vi "Read Class Path.vi"(8 "error in (no error)":errorcluster, 11 "Open Form in":refnum<class "Open Form.lvclass">) -> (0 "error out":errorcluster, 2 "Class Path":path, 3 "Open Form out":refnum<class "Open Form.lvclass">)   [LabVIEW 2020, in "Open Form.lvclass"]
uses:
  Open Form.lvclass
  Open Form.lvclass/Open Form.ctl
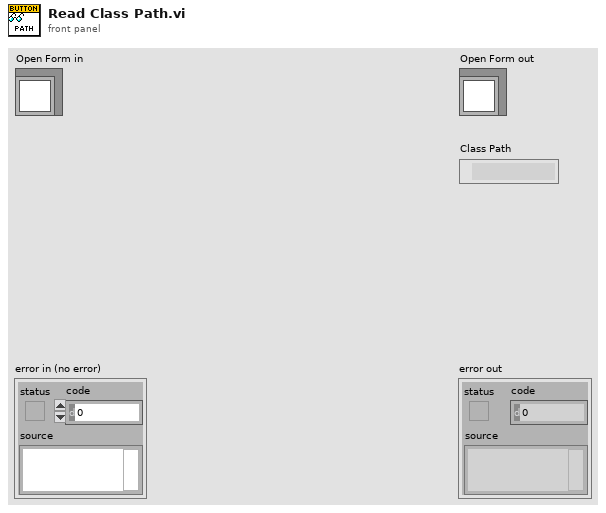
[diagram p1: front panel]
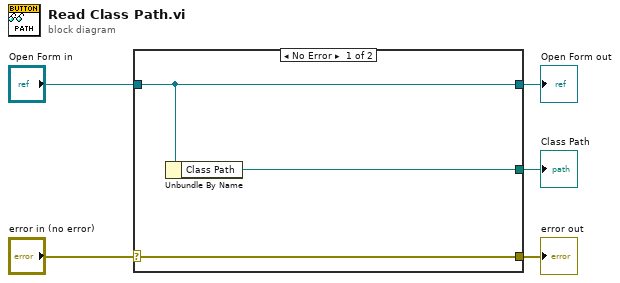
[diagram p0: block diagram]
diagram:
  n1 = case shown="No Error" "error in (no error)" {
    selector: "error in (no error)" -> [w8 w9]
    tunnel: [w8 w9] -> w4
    tunnel: [w7 w10] -> w2
    tunnel: "Open Form in" -> [w7 w10]
    tunnel: [w6 _] -> w1
    frame No Error {
      n2 = Unbundle By Name(w7) -> ("Class Path"=w6:path)
    }
    frame Error {
    }
  }
  "error out" <- w4
  "Open Form out" <- w2
  "Class Path" <- w1
